vi "G#RemoteProxy_GetAttributes.vi"(0 "reference in":refnum<class "G#RemoteProxy.lvclass">, 1 "return data? (T)":bool=TRUE, 5 "error in (no error)":errorcluster) -> (14 "reference out":refnum<class "G#RemoteProxy.lvclass">, 15 "attributes ref":T3, 16 "attributes":T1, 19 "error out":errorcluster)   [LabVIEW 2017, in "G#RemoteProxy.lvclass"]
doc: "Returns a reference and if wanted the actual data values of the attributes. This method is used by the subclasses to access parent attributes."
uses:
  <vilib>/addons/_AddQ/G#Debugger/G#RemoteProxy/G#RemoteProxy.lvclass
  <vilib>/addons/_AddQ/G#Debugger/G#RemoteProxy/utils/ObjectAttributesRef.ctl
  <vilib>/addons/_AddQ/G#Debugger/G#RemoteProxy/protected/ObjectAttributesProxy.ctl
  <vilib>/addons/_AddQ/G#Object/utils/G#Object_ClassHierarchy.ctl
  <vilib>/addons/_AddQ/G#Object/G#Object.lvclass
  <vilib>/addons/_AddQ/G#Debugger/G#RemoteProxy/G#RemoteProxy.lvclass/G#RemoteProxy.ctl
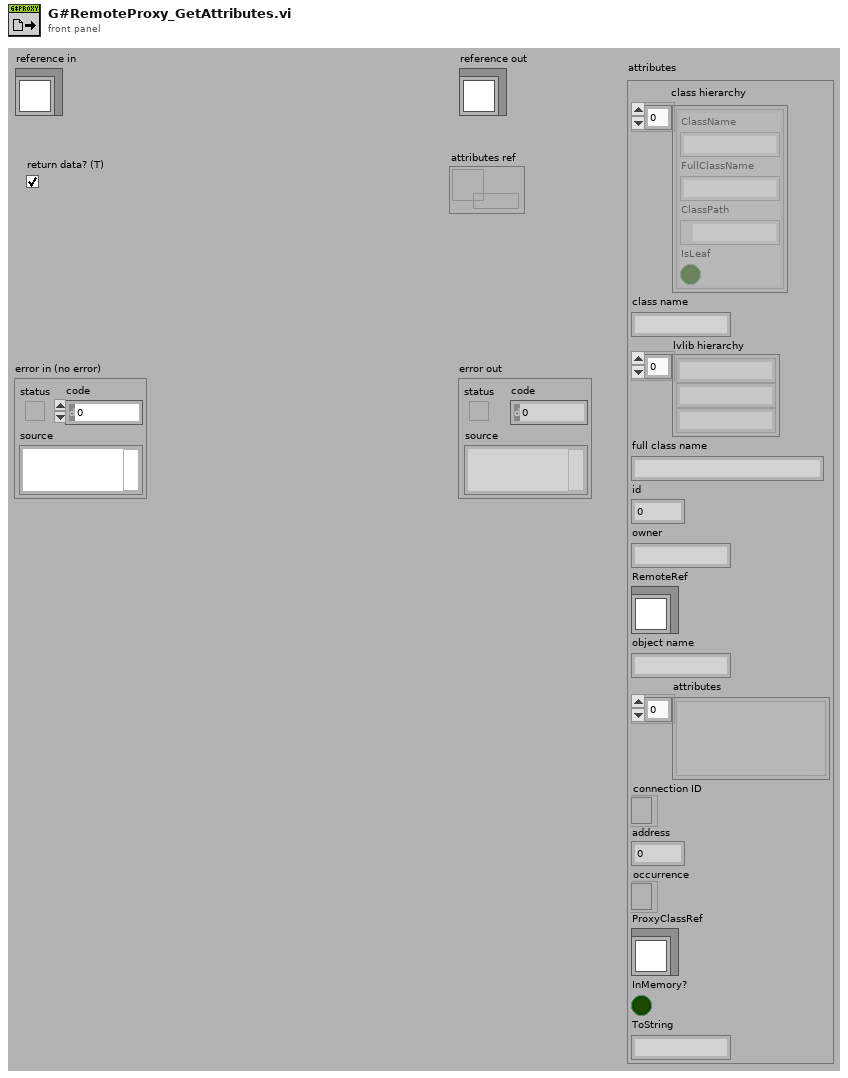
[diagram p1: front panel]
types:
  T1 = typedef "G#RemoteProxy.lvclass/ObjectAttributesProxy.ctl" = cluster{"class hierarchy":T2[], "class name":string, "lvlib hierarchy":string[], "full class name":string, "id":u32, "owner":string, "RemoteRef":refnum<class "G#Object.lvclass">, "object name":string, "attributes":variant[], "connection ID":refnum<k5>, "address":u32, "occurrence":refnum<k4>, "ProxyClassRef":refnum<class "G#RemoteProxy.lvclass">, "InMemory?":bool, "ToString":string}
  T2 = typedef "G#Object.lvclass/G#Object_ClassHierarchy.ctl" = cluster{"ClassName":string, "FullClassName":string, "ClassPath":path, "IsLeaf":bool}
  T3 = typedef "G#RemoteProxy.lvclass/ObjectAttributesRef.ctl" = refnum<data-value>
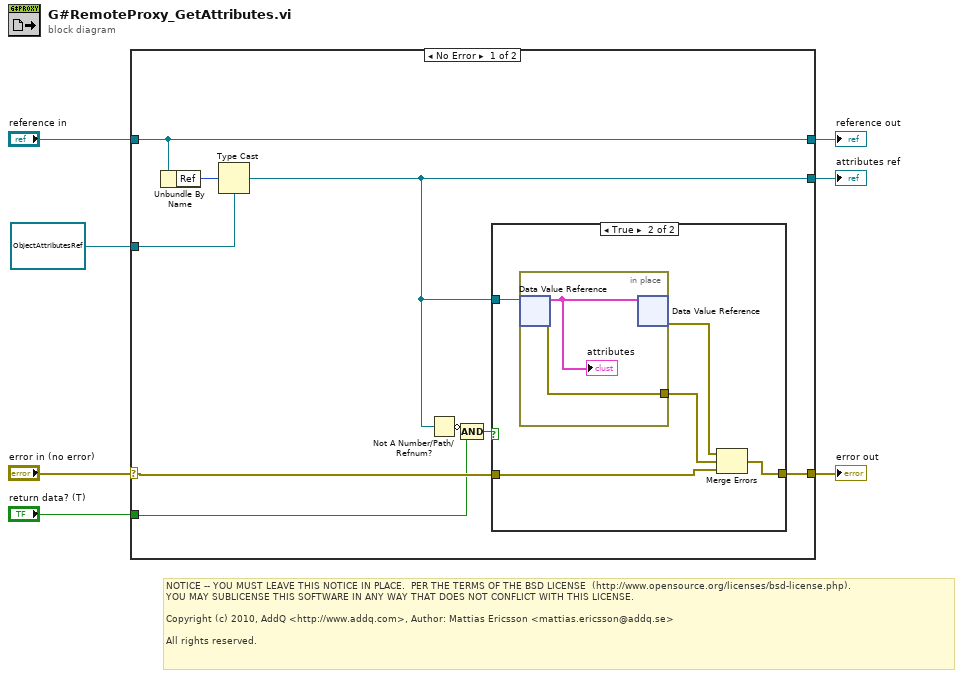
[diagram p0: block diagram]
diagram:
  # "NOTICE -- YOU MUST LEAVE THIS NOTICE IN PLACE.  PER THE TERMS OF THE BSD LICENSE  (http://www.opensource.org/licenses/bsd-license.php).\nYOU MAY SUBLICENSE THIS SOFTWARE IN ANY WAY THAT DOES NOT CONFLICT WITH THIS LICENSE.\n\nCopyright (c) 2010, AddQ <http://www.addq.com>, Author: Mattias Ericsson <mattias.ericsson@addq.se>\n\nAll rights reserved."
  n1 = case shown="No Error" "error in (no error)" {
    selector: "error in (no error)" -> [w12 w27]
    tunnel: [w16 w27] -> w6
    tunnel: [w13 w26] -> w4
    tunnel: "reference in" -> [w13 w26]
    tunnel: [w11 w25] -> w3
    tunnel: "return data? (T)" -> [w9 _]
    tunnel: T3 refnum ("attributes ref") -> [w14 w25]
    frame No Error {
      n2 = Unbundle By Name(w13) -> ("Ref"=w15:u32)
      n3 = Type Cast(type=w14, x=w15) -> (*(type *) &x=w11:T3)
      n4 = Not A Number/Path/Refnum?(number/path/refnum=w11) -> (NaN/Path/Refnum?=w10:bool)
      n5 = Compound Arithmetic op=AND(invert w10, w9) -> (w8:bool)
      n6 = case shown="True" w8 {
        tunnel: w11 -> [_ w22]
        tunnel: w12 -> [w17 w21]
        tunnel: [w17 w18] -> w16
        frame False {
        }
        frame True {
          n7 = in-place {
            in-place-border: [w24] -> w20
            n8 = in-place-dvr #1(w22) -> (w23:T1, w24:errorcluster)
            "attributes" <- w23
            n9 = in-place-dvr #1(w23) -> (w19:errorcluster)  [unwired: 1 out]
          }
          n10 = Merge Errors(w19, w20, w21) -> (w18:errorcluster)
        }
      }
    }
    frame Error {
    }
  }
  "error out" <- w6
  "reference out" <- w4
  "attributes ref" <- w3
